vi "Test Finding Tests at Empty Path Finds all Test In App Instance.vi"(8 "error in (no error)":errorcluster, 11 "Test Finder Test in":refnum<class "Finder Test.lvclass">) -> (0 "error out":errorcluster, 3 "Test Finder Test out":refnum<class "Finder Test.lvclass">)   [LabVIEW 2020, in "LUnit Tests.lvlib" / "Finder Test.lvclass"]
uses:
  Finder Test.lvclass
  source/Framework/Helper Classes/Test Finder/Test Finder.lvclass
  ab21dd14-79cd-4872-adbc-04192090847d.vi
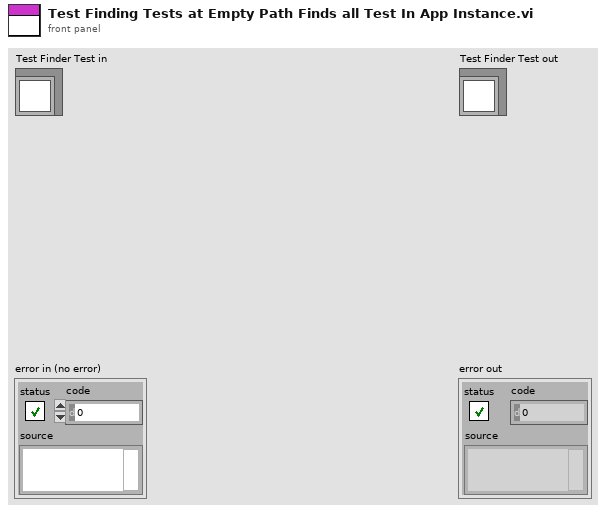
[diagram p1: front panel]
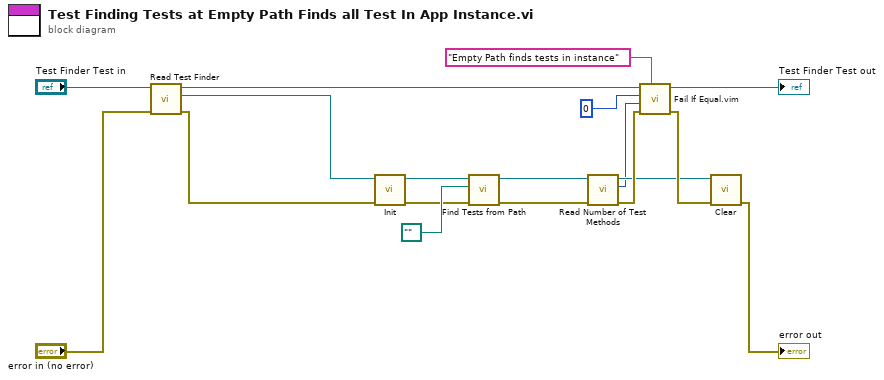
[diagram p0: block diagram]
diagram:
  n1 = call "Read Test Finder.vi"("error in (no error)"="error in (no error)", "Test Finder In"="Test Finder Test in") -> ("error out"=w9:errorcluster, "Test Finder.lvclass"=w10:refnum<class "Test Finder.lvclass">, "Test Finder Out"=w16:refnum<class "Finder Test.lvclass">)  [unwired: 7 in]
  n2 = call-dynamic "Init.vi"("error in (no error)"=w9, "Test Finder in"=w10) -> ("error out"=w11:errorcluster, "Test Finder out"=w12:refnum<class "Test Finder.lvclass">)  [unwired: 8 in]
  n3 = call-dynamic "Find Tests from Path.vi"("error in (no error)"=w11, "Project or Class Path"=path "", "Test Case Finder In"=w12) -> ("error out"=w5:errorcluster, "Test Case Finder Out"=w4:refnum<class "Test Finder.lvclass">)  [unwired: 7 in]
  n4 = call "Read Number of Test Methods.vi"("error in (no error)"=w5, "Test Finder In"=w4) -> ("error out"=w6:errorcluster, "Number of Test Methods found"=w2:i32, "Test Finder Out"=w3:refnum<class "Test Finder.lvclass">)  [unwired: 7 in]
  n5 = call "Fail If Equal.vim"("Description"="Empty Path finds tests in instance", "error in (no error)"=w6, "Actual"=w2, "Expected"=0 ("Number of Test Methods found"), "LUnit Test Case In"=w16) -> ("error out"=w8:errorcluster, "LUnit Test Case Out"=→"Test Finder Test out":refnum<class "Finder Test.lvclass">)  [unwired: 5 in]
  n6 = call "Clear.vi"("error in (no error)"=w8, "Test Finder in"=w3) -> ("error out"=→"error out":errorcluster)  [unwired: 8 in, 1 out]
